vi "Upload program temp.vi"(7 "Address":dbl=1.0, 8 "error in (no error)":errorcluster, 9 "Segment":dbl=6.0, 10 "Temp":dbl=1000.0, 11 "VISA resource name (IN)":refnum<visa-resource-name>) -> (0 "error out":errorcluster, 3 "VISA resource name (OUT)":refnum<visa-resource-name>)   [LabVIEW 2010, in "Yudian AI508.lvlib"]
doc: "Use this template to build a VI to use as a subVI."
uses:
  <instrlib>/Yudian AI508/Yudian AI508.lvlib
panel:
  out "Recieved Raw Data":string
  out "Recevied Temp.  data":dbl
  out "Data buffer":string
  out "Digital shift":i32
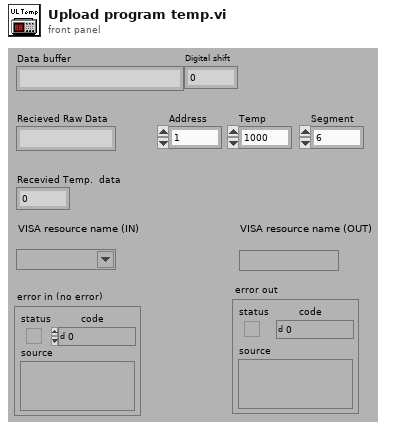
[diagram p1: front panel]
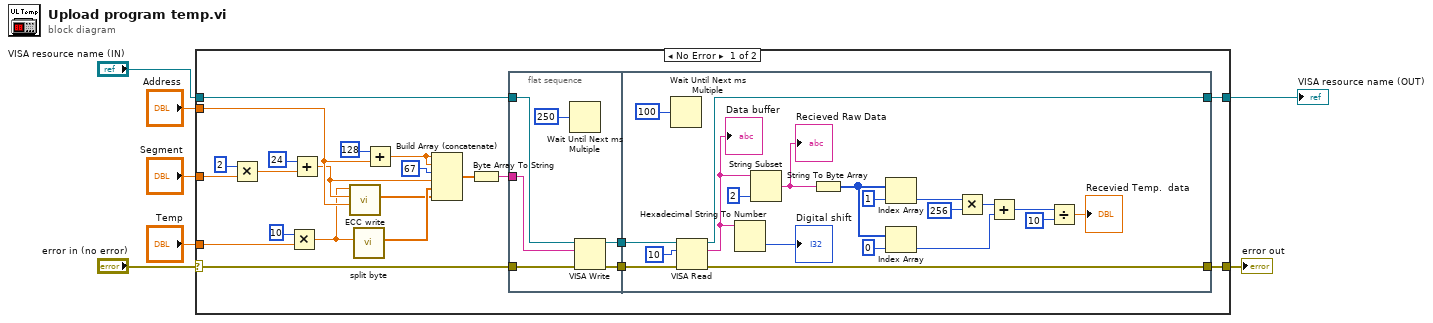
[diagram p0: block diagram]
diagram:
  n1 = case shown="No Error" "error in (no error)" {
    selector: "error in (no error)" -> [w24 w57]
    tunnel: [w26 w57] -> w7
    tunnel: [w27 w56] -> w6
    tunnel: "VISA resource name (IN)" -> [w25 w56]
    tunnel: "Address" -> [w17 _]
    tunnel: "Segment" -> [w13 _]
    tunnel: "Temp" -> [w9 _]
    frame No Error {
      n2 = Multiply(x=2, y=w13) -> (x*y=w11:dbl)
      n3 = Multiply(x=10, y=w9) -> (x*y=w10:dbl)
      n4 = Add(x=24, y=w11) -> (x+y=w14:dbl)
      n5 = call <instrlib>:"ECC write.vi"("Address"=w17, "Parameter code"=w14, "Value"=w10) -> ("Data array"=w16:dbl[])  [unwired: 8 in]
      n6 = call <instrlib>:"split byte.vi"("Value"=w10) -> ("Array"=w18:dbl[])  [unwired: 10 in]
      n7 = Add(x=128, y=w17) -> (x+y=w23:dbl)
      n8 = Build Array (concatenate)(w23, w23, 67, w14, w18, w16) -> (w20:dbl[])
      n9 = Byte Array To String(unsigned byte array=w20) -> (string=w19:string)
      n10 = flat-sequence {
        tunnel: w24 -> [w35]
        tunnel: w25 -> [w32]
        tunnel: [w34] -> w29
        tunnel: [w33] -> w28
        tunnel: w19 -> [w30]
        tunnel: w29 -> [w41]
        tunnel: w28 -> [w40]
        tunnel: [w38] -> w27
        tunnel: [w37] -> w26
        frame #0 {
          n11 = Wait Until Next ms Multiple(millisecond multiple=250) -> ()  [unwired: 1 out]
          n12 = VISA Write(VISA resource name=w32, write buffer=w30, error in (no error)=w35) -> (VISA resource name out=w33:refnum<visa-resource-name>, error out=w34:errorcluster)  [unwired: 1 out]
        }
        frame #1 {
          n13 = Wait Until Next ms Multiple(millisecond multiple=100) -> ()  [unwired: 1 out]
          n14 = VISA Read(VISA resource name=w40, byte count=u32 10 ("字节总数"), error in (no error)=w41) -> (VISA resource name out=w38:refnum<visa-resource-name>, read buffer=w43:string, error out=w37:errorcluster)  [unwired: 1 out]
          "Data buffer" <- w43
          n15 = Hexadecimal String To Number(string=w43) -> (number=→"Digital shift":u32)  [unwired: 3 out]
          n16 = String Subset(string=w43, length (rest)=2 ("length (rest)")) -> (substring=w53:string)  [unwired: 1 out]
          "Recieved Raw Data" <- w53
          n17 = String To Byte Array(string=w53) -> (unsigned byte array=w51:u8[])
          n18 = Index Array(array=w51, index=1) -> (element=w50:u8)
          n19 = Index Array(array=w51, index=0) -> (element=w47:u8)
          n20 = Multiply(x=w50, y=u16 256) -> (x*y=w48:u16)
          n21 = Add(x=w48, y=w47) -> (x+y=w46:u16)
          n22 = Divide(x=w46, y=u16 10) -> (x/y=→"Recevied Temp.  data":dbl)
        }
      }
    }
    frame Error {
    }
  }
  "error out" <- w7
  "VISA resource name (OUT)" <- w6
